vi "Low Pass Filter subVI.vi"(8 "error in (no error)":errorcluster, 9 "Element Data":u16, 10 "Array":waveform(dbl)[](array[waveform]), 11 "Lockin.DAQ in":refnum<class "Instrument.DAQ.lvclass">) -> (0 "error out":errorcluster, 1 "Fc (Hz)":dbl, 2 "signal out":waveform(dbl)[](array[waveform]))   [LabVIEW 2019, in "Instrument.DAQ.lvclass"]
uses:
  Instrument.DAQ.lvclass
  Instrument.DAQ.lvclass/Instrument.DAQ.ctl
  <vilib>/addons/Digital Filter Design/Process.llb/DFD Filtering (Wfm NChan).vi
  <vilib>/addons/Digital Filter Design/NI_DigFilterLicensed.lvlib
panel:
  out "Lockin.DAQ out":refnum<class "Instrument.DAQ.lvclass">
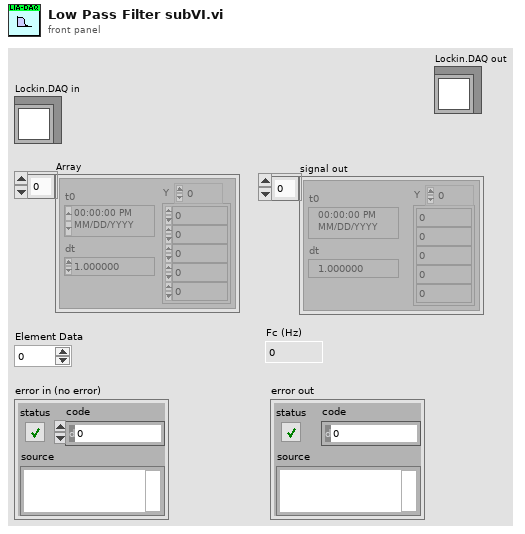
[diagram p1: front panel]
types:
  T1 = enum16{"Lowpass", "Highpass", "Bandpass", "Bandstop"}
  T2 = typedef "Instrument.DAQ.lvclass/REF-cluster.ctl" = T3[]
  T3 = typedef "Instrument UI.Lockin.lvclass/REF Channel--Cluster.ctl" = cluster{"Enable?":bool, "Channel":i32, "Frequency":dbl, "Phase":dbl, "TC":dbl, "Roll-Off":i32}
  T4 = typedef "NI_DigFilterLicensed.lvlib/DFD Filter Obj.ctl" = cluster{"mSRate_Fs":dbl, "mSRate_Version":string, "mSRate_Comments":string, "mSRate_OrgCoef":T5, "mSRate_CurCoef":T5, "mSRate_Quantized?":bool, "mSRate_QCoef":T5, "mSRate_QSettings":T7[], "mSRate_Order":i32, "mSRate_Scaling":cluster{"mSRate_ScaleByPowerOf2?":bool, "mSRate_ScaleType":T9}}
  T5 = typedef "NI_DigFilterLicensed.lvlib/DFD Filter Coef.ctl" = cluster{"type":T6, "gain":dbl, "coef a (k)":dbl[], "coef b (v)":dbl[]}
  T6 = typedef "NI_DigFilterLicensed.lvlib/DFD Filter Structure Type Selector.ctl" = enum16{"Undefined", "FIR Direct Form", "FIR Direct Form Transposed", "FIR Symmetric", "FIR Antisymmetric", "IIR Direct Form I", "IIR Direct Form I Transposed", "IIR Direct Form II", "IIR Direct Form II Transposed", "IIR Cascaded Second Order Sections Form I", "IIR Cascaded Second Order Sections Form I Transposed", "IIR Cascaded Second Order Sections Form II", "IIR Cascaded Second Order Sections Form II Transposed", "Lattice Allpass (basic sections)", "Lattice Allpass (one multiplier sections)", "Lattice Allpass (normalized sections)", "Lattice AR (basic sections)", "Lattice AR (one multiplier sections)", "Lattice AR (normalized sections)", "Lattice MA (minimum phase)", "Lattice MA (maximum phase)", "Lattice ARMA (basic sections)", "Lattice ARMA (one multiplier sections)", "Lattice ARMA (normalized sections)"}
  T7 = typedef "NI_DigFilterLicensed.lvlib/dfd_Internal Quantization Settings.ctl" = cluster{"source":T8, "wl":i16, "iwl":i16, "overflow mode":enum16{"Saturation", "Wrap"}, "rounding mode":enum16{"Nearest", "Truncation"}, "signed?":bool}
  T8 = typedef "NI_DigFilterLicensed.lvlib/dfd_Internal Quantization Srcs.ctl" = u16
  T9 = typedef "NI_DigFilterLicensed.lvlib/DFD Coef Norm Type.ctl" = enum16{"No Norm", "Time Domain 1-Norm", "Time Domain 2-Norm", "Time Domain Inf-Norm"}
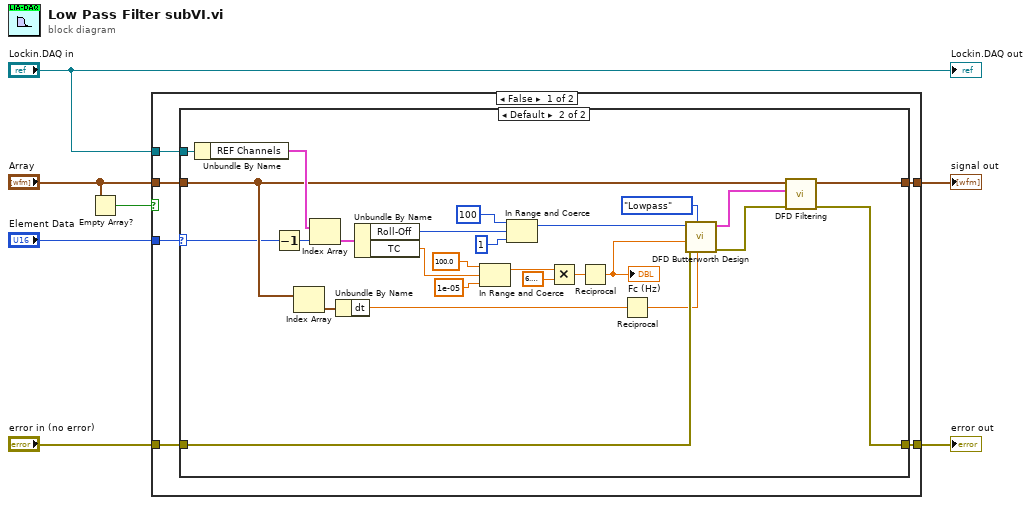
[diagram p0: block diagram]
diagram:
  n1 = Empty Array?(array="Array") -> (empty?=w1:bool)
  n2 = case shown="False" w1 {
    tunnel: "error in (no error)" -> [w13 w43]
    tunnel: [w12 w43] -> w6
    tunnel: [w11 w42] -> w5
    tunnel: "Lockin.DAQ in" -> [w10 _]
    tunnel: "Element Data" -> [w8 _]
    tunnel: "Array" -> [w9 w42]
    frame False {
      n3 = case shown="Default" w8 {
        selector: w8 -> [_ w16]
        tunnel: w13 -> [w15 w41]
        tunnel: [w15 w40] -> w12
        tunnel: w9 -> [w14 w38]
        tunnel: [w14 w18] -> w11
        tunnel: w10 -> [_ w17]
        frame 0 {
        }
        frame Default {
          n4 = Unbundle By Name(w17) -> ("REF Channels"=w39:T2)
          n5 = Decrement(x=w16) -> (x-1=w29:u16)
          n6 = Index Array(array=w38) -> (element=w36:waveform(dbl))  [unwired: 1 in]
          n7 = Index Array(array=w39, index=w29) -> (element=w33:T3)
          n8 = Unbundle By Name(w36) -> ("dt"=w35:dbl)
          n9 = Unbundle By Name(w33) -> ("Roll-Off"=w31:i32, "TC"=w32:dbl)
          n10 = In Range and Coerce(upper limit=100.0, x=w32, lower limit=1e-05) -> (coerced(x)=w21:dbl)  [unwired: 1 out]
          n11 = In Range and Coerce(upper limit=100, x=w31, lower limit=1) -> (coerced(x)=w19:i32)  [unwired: 1 out]
          n12 = Multiply(x=w21, y=6.283185307179586) -> (x*y=w25:dbl)
          n13 = Reciprocal(x=w25) -> (1/x=w28:dbl)
          "Fc (Hz)" <- w28
          n14 = Reciprocal(x=w35) -> (1/x=w27:dbl)
          n15 = call <vilib>:"DFD Butterworth Design.vi"("fs [Hz]"=w27, "filter type"=T1."Lowpass", "error in (no error)"=w41, "low cutoff freq [Hz]"=w28, "order"=w19) -> ("error out"=w37:errorcluster, "filter out"=w34:T4)  [unwired: 5 in]
          n16 = call-poly <vilib>:"DFD Filtering.vi"("error in (no error)"=w37, "filter"=w34, "signal in"=w38) -> ("error out"=w40:errorcluster, "signal out"=w18:waveform(dbl)[])  [unwired: 7 in]
        }
      }
    }
    frame True {
    }
  }
  "error out" <- w6
  "signal out" <- w5
  "Lockin.DAQ out" <- "Lockin.DAQ in"
